vi "12.2-2 ParticleSeperate.vi"() -> ()   [LabVIEW 2016]
doc: "This example shows how to use the Edge Tool in NI Vision. The Edge Tool finds edges (or sharp transitions in the pixels values) along a given line or ROI profile. The Edge Tool is a precursor function to many of the gauging and inspection tasks. For example, the location of the edges found along a line profile across an object can interpreted as the boundaries of the object whose dimensions have to be measured for a gauging application or the presence of a crack in the surface of an object for an inspection application."
uses:
  <vilib>/vision/NI_Vision_Development_Module.lvlib
panel:
  out "Seperated":T1(plugin-control)
  out "Src":T1(plugin-control)
  in  "Structuring Element":i32[][](array[numeric])=[[0, 1, 0], [1, 1, 1], [0, 0, 0]]
  in  "Hexa Pixel?":bool
  in  "# of iterations":i32=4
  in  "Operation":u16(ring)=3 items=["AutoM", "Close", "Dilate", "Erode", "Gradient", "Gradient out", "Gradient in", "Hit miss", "Open", "PClose", "POpen", "Thick", "Thin"]
  out "Erode(Nb of Erode=4)":T1(plugin-control)
  in  "Stop":bool
  # "Instructions:\n1) Run VI and change the \"# of iterations\";\n2) Check the display of \"Erode\" and \"Seperated\" when # of iterations is 3 and 4;\n3) Notice that the particles will be seperated when # of \niterations is 4."
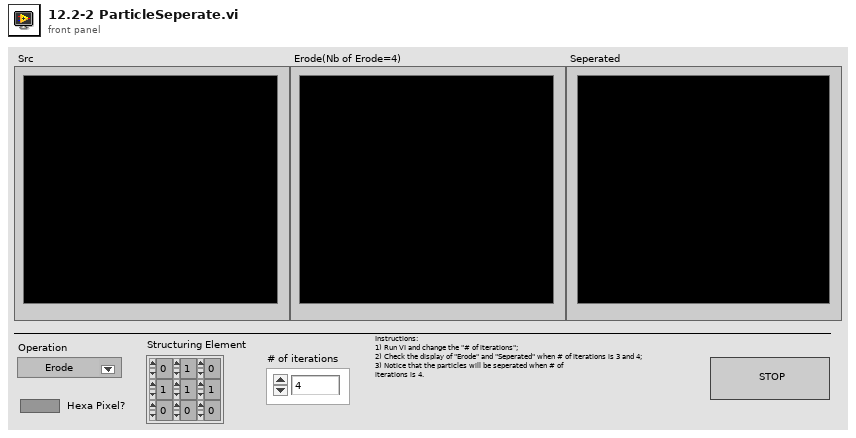
[diagram p1: front panel]
types:
  T1 = typedef "IMAQ Image.ctl" = refnum<image>
  T2 = cluster{"Hexa Pixel?":bool, "Operation":u16, "Structuring Element":i32[][], "# of iterations":i32}
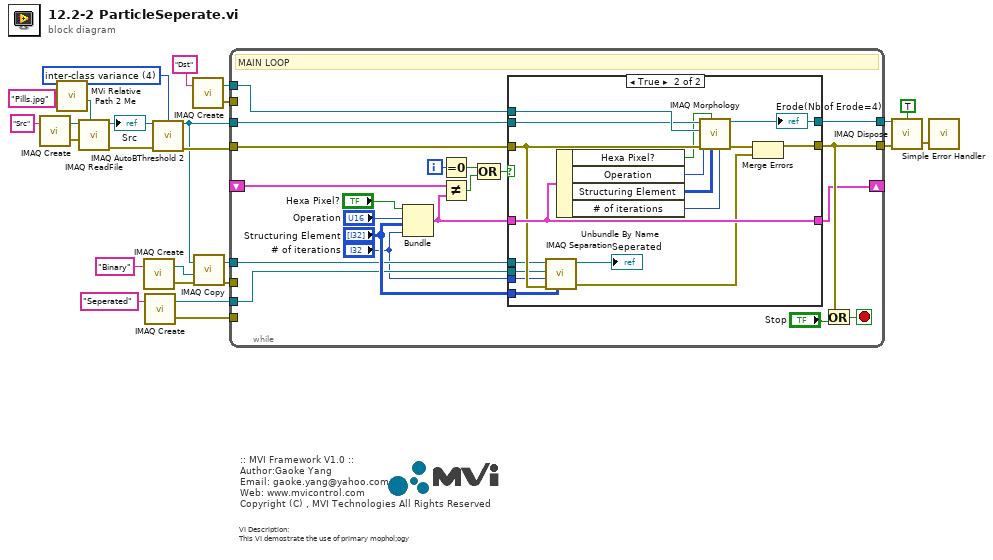
[diagram p0: block diagram]
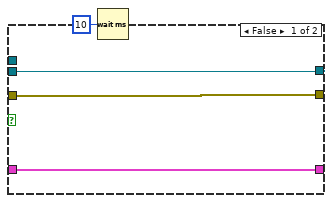
[diagram p2: hidden frame]
diagram:
  w16 = 4 items=["clustering", "entropy", "metric", "moments", "inter-class variance"] ("Method")
  # "VI Description:\nThis VI demostrate the use of primary mophol;ogy"
  # ":: MVI Framework V1.0 ::\nAuthor:Gaoke Yang\nEmail: gaoke.yang@yahoo.com\nWeb: www.mvicontrol.com\nCopyright (C) , MVI Technologies All Rights Reserved"
  n1 = call "IMAQ Create"("Image Name"="Src") -> ("New Image"=w24:T1, "error out"=w23:errorcluster)  [unwired: 4 in]
  n2 = call "MVi Relative Path 2 Me.vi"("Relative Path"="Pills.jpg" ("name or relative path")) -> ("Appended Dir"=w19:path)  [unwired: 5 in, 1 out]
  n3 = call "IMAQ ReadFile"("File Path"=w19, "error in (no error)"=w23, "Image"=w24) -> ("error out"=w14:errorcluster, "Image Out"=w13:T1)  [unwired: 4 in, 3 out]
  "Src" <- w13
  n4 = call "IMAQ Create"("Image Name"="Binary") -> ("New Image"=w5:T1, "error out"=w6:errorcluster)  [unwired: 4 in]
  n5 = call "IMAQ Create"("Image Name"="Seperated") -> ("New Image"=w1:T1, "error out"=w2:errorcluster)  [unwired: 4 in]
  n6 = call "IMAQ AutoBThreshold 2"("Image Src"=w13, "Method (clustering)"=w16, "error in (no error)"=w14) -> ("Image Dst Out"=w4:T1, "error out"=w15:errorcluster)  [unwired: 5 in, 6 out]
  n7 = call "IMAQ Create"("Image Name"="Dst") -> ("New Image"=w11:T1, "error out"=w10:errorcluster)  [unwired: 4 in]
  n8 = call "IMAQ Copy"("error in (no error)"=w6, "Image Dst"=w5, "Image Src"=w4) -> ("error out"=w8:errorcluster, "Image Dst Out"=w7:T1)  [unwired: 3 in]
  n9 = while "MAIN LOOP" {
    tunnel: w4 -> [w44]
    tunnel: w15 -> [w45]
    tunnel: [w40] -> w22
    tunnel: [w41] -> w21
    shift-right: [w37] -> _
    shift-left: _ -> [w34]
    tunnel: w11 -> [w31]
    tunnel: w10 -> [_]
    tunnel: w8 -> [_]
    tunnel: w7 -> [w29]
    tunnel: w2 -> [_]
    tunnel: w1 -> [w28]
    i -> [w39]
    stop <- w42 stop-if-true
    # "MAIN LOOP"
    n10 = Bundle("Hexa Pixel?"="Hexa Pixel?", "Operation"="Operation", "Structuring Element"="Structuring Element", "# of iterations"="# of iterations") -> (w35:T2)  [unwired: 1 in]
    n11 = Equal To 0?(x=w39) -> (x = 0?=w36:bool)
    n12 = Not Equal?(x=w34, y=w35) -> (x != y?=w33:bool)
    n13 = Compound Arithmetic op=OR(w36, w33) -> (w38:bool)
    n14 = case shown="True" w38 {
      tunnel: w45 -> [w48 w62]
      tunnel: w44 -> [w49 w60]
      tunnel: [w49 w52] -> w41
      tunnel: [w48 w58] -> w40
      tunnel: [w46 w65] -> w37
      tunnel: w35 -> [w46 w65]
      tunnel: w31 -> [_ w66]
      tunnel: "Structuring Element" -> [_ w61]
      tunnel: "# of iterations" -> [_ w59]
      tunnel: w29 -> [_ w57]
      tunnel: w28 -> [_ w56]
      frame False {
        n15 = Wait (ms)(milliseconds to wait=u32 10) -> ()  [unwired: 1 out]
      }
      frame True {
        n16 = call "IMAQ Separation"("Structuring Element"=w61, "error in (no error)"=w62, "Nb of Erosion"=w59, "Image Dst"=w56, "Image Src"=w57) -> ("error out"=w51:errorcluster, "Image Dst Out"=→"Seperated":T1)  [unwired: 5 in]
        n17 = Unbundle By Name(w65) -> ("Hexa Pixel?"=w54:bool, "Operation"=w63:u16, "Structuring Element"=w64:i32[][], "# of iterations"=w55:i32)
        n18 = call "IMAQ Morphology"("Number of iterations (1)"=w55, "Structuring Element"=w64, "Square/Hexa (Square)"=w54, "error in (no error)"=w62, "Operation"=w63, "Image Dst"=w66, "Image Src"=w60) -> ("error out"=w53:errorcluster, "Image Dst Out"=w52:T1)  [unwired: 3 in]
        "Erode(Nb of Erode=4)" <- w52
        n19 = Merge Errors(w53, w51) -> (w58:errorcluster)
      }
    }
    n20 = Or(x=w40, y="Stop") -> (x .or. y?=w42:bool)
  }
  n21 = call "IMAQ Dispose"("All Images? (No)"=TRUE, "Image"=w21, "error in (no error)"=w22) -> ("error out"=w18:errorcluster)  [unwired: 3 in]
  n22 = call <vilib>:"Simple Error Handler.vi"("error in (no error)"=w18) -> ()  [unwired: 4 in, 5 out]
